vi "Ejercicio 1.2.10.vi"() -> ()   [LabVIEW 2013]
panel:
  out "Boolean 2":bool
  in  "Boolean":bool
  in  "String 2":string
  out "String":string
  in  "Numeric 4":i32
  out "Numeric 3":i32
  out "Numeric 2":dbl
  in  "Numeric":dbl
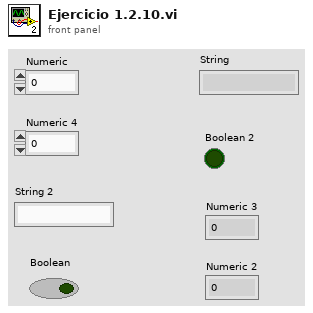
[diagram p1: front panel]
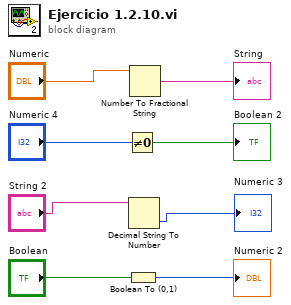
[diagram p0: block diagram]
diagram:
  n1 = Not Equal To 0?(x="Numeric 4") -> (x != 0?=→"Boolean 2":bool)
  n2 = Boolean To (0,1)(Boolean="Boolean") -> (0, 1=→"Numeric 2":i16)
  n3 = Decimal String To Number(string="String 2") -> (number=→"Numeric 3":i32)  [unwired: 2 in, 1 out]
  n4 = Number To Fractional String(number="Numeric") -> (F-format string=→"String":string)  [unwired: 3 in]
